vi "Get Database Items.vi"(6 "bookable":bool, 7 "search string":string, 8 "error in (no error)":errorcluster, 9 "offset (0)":u32, 10 "limit (15)":u32=15, 11 "eLab in":refnum<class "PL eLabFTW Client.lvclass">) -> (0 "error out":errorcluster, 2 "database items":T1(array[cluster]) {"last comment"."datetime" format="%<%X\n%x>T"; "last change"."datetime" format="%<%X\n%x>T"; "start datetime" format="%<%X\n%x>T"}, 3 "eLab out":refnum<class "PL eLabFTW Client.lvclass">)   [LabVIEW 2015, in "PL eLabFTW Client.lvclass"]
doc: "Gets database items. Limit, offset and search string can be used to narrow down the output."
uses:
  PL eLabFTW Client.lvclass
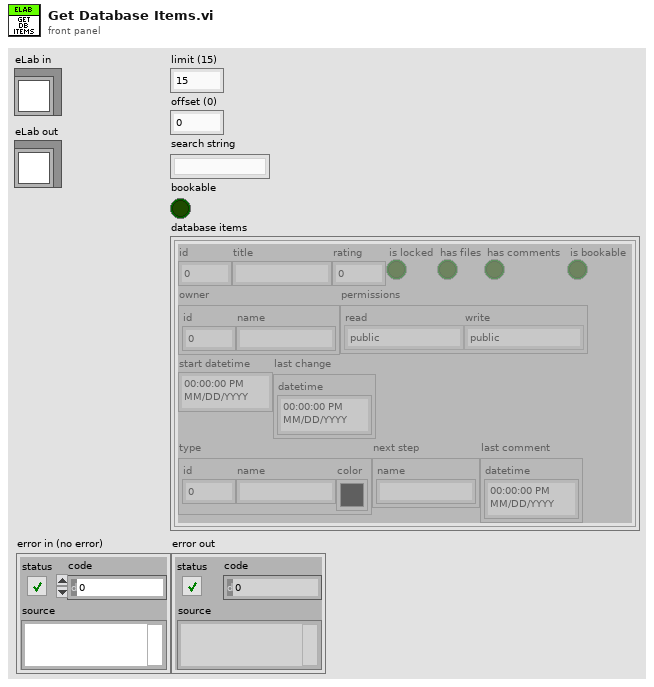
[diagram p1: front panel]
types:
  T1 = cluster{"id":u32, "title":string, "rating":u32, "is locked":bool, "has files":bool, "has comments":bool, "is bookable":bool, "owner":cluster{"id":u32, "name":string}, "permissions":cluster{"read":enum16{"public", "organization", "team", "owner and admins", "owner"}, "write":enum16{"public", "organization", "team", "owner and admins", "owner"}}, "start datetime":timestamp, "last change":cluster{"datetime":timestamp}, "type":cluster{"id":u32, "name":string, "color":u32}, "next step":cluster{"name":string}, "last comment":cluster{"datetime":timestamp}}[]
  T2 = cluster{"id":string, "title":string, "date":string, "category":string, "rating":string, "userid":string, "locked":string, "canread":string, "canwrite":string, "lastchange":string, "up_item_id":string, "has_attachment":string, "next_step":string, "category_id":string, "color":string, "fullname":string, "recent_comment":string, "has_comment":string, "bookable":string}[]
  T3 = cluster{"id":u32, "title":string, "rating":u32, "is locked":bool, "has files":bool, "has comments":bool, "is bookable":bool, "owner":cluster{"id":u32, "name":string}, "permissions":cluster{"read":enum16{"public", "organization", "team", "owner and admins", "owner"}, "write":enum16{"public", "organization", "team", "owner and admins", "owner"}}, "start datetime":timestamp, "last change":cluster{"datetime":timestamp}, "type":cluster{"id":u32, "name":string, "color":u32}, "next step":cluster{"name":string}, "last comment":cluster{"datetime":timestamp}}
  T4 = enum16{"public", "organization", "team", "owner and admins", "owner"}
  T5 = cluster{"id":i32, "title":i32, "date":i32, "category":i32, "rating":i32, "userid":i32, "locked":i32, "canread":i32, "canwrite":i32, "lastchange":i32, "up_item_id":i32, "has_attachment":i32, "next_step":i32, "category_id":i32, "color":i32, "fullname":i32, "recent_comment":i32, "has_comment":i32, "bookable":i32}
  T6 = cluster{"id":bool, "title":bool, "date":bool, "category":bool, "rating":bool, "userid":bool, "locked":bool, "canread":bool, "canwrite":bool, "lastchange":bool, "up_item_id":bool, "has_attachment":bool, "next_step":bool, "category_id":bool, "color":bool, "fullname":bool, "recent_comment":bool, "has_comment":bool, "bookable":bool}
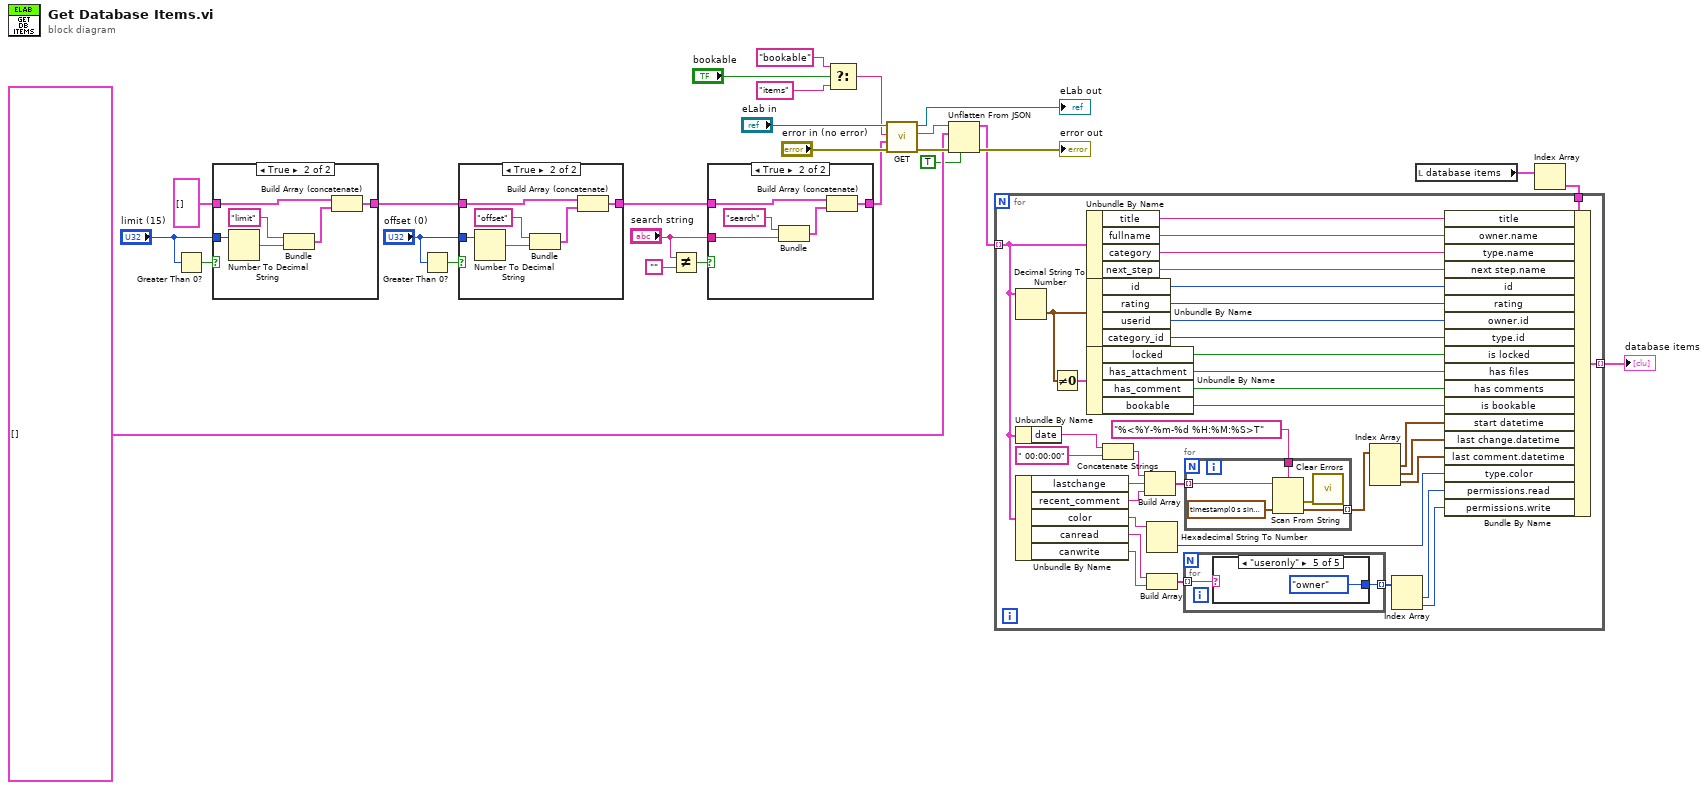
[diagram p0: block diagram]
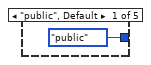
[diagram p2: hidden frame]
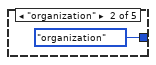
[diagram p3: hidden frame]
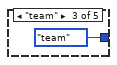
[diagram p4: hidden frame]
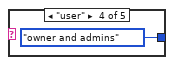
[diagram p5: hidden frame]
diagram:
  n1 = Greater Than 0?(x="limit (15)") -> (x > 0?=w21:bool)
  n2 = case shown="True" w21 {
    tunnel: "limit (15)" -> [_ w34]
    tunnel: [w28 w30] -> w16
    tunnel: cluster{string, string}[] [] -> [w28 w29]
    frame False {
    }
    frame True {
      n3 = Number To Decimal String(number=w34) -> (decimal integer string=w33:string)  [unwired: 1 in]
      n4 = Bundle("limit", w33) -> (w31:cluster{string, string})  [unwired: 1 in]
      n5 = Build Array (concatenate)(w29, w31) -> (w30:cluster{string, string}[])
    }
  }
  n6 = Greater Than 0?(x="offset (0)") -> (x > 0?=w18:bool)
  n7 = case shown="True" w18 {
    tunnel: "offset (0)" -> [_ w41]
    tunnel: [w35 w37] -> w14
    tunnel: w16 -> [w35 w36]
    frame False {
    }
    frame True {
      n8 = Number To Decimal String(number=w41) -> (decimal integer string=w40:string)  [unwired: 1 in]
      n9 = Bundle("offset", w40) -> (w38:cluster{string, string})  [unwired: 1 in]
      n10 = Build Array (concatenate)(w36, w38) -> (w37:cluster{string, string}[])
    }
  }
  n11 = Not Equal?(x="search string", y="") -> (x != y?=w15:bool)
  n12 = case shown="True" w15 {
    tunnel: "search string" -> [_ w43]
    tunnel: [w42 w45] -> w10
    tunnel: w14 -> [w42 w44]
    frame False {
    }
    frame True {
      n13 = Bundle("search", "search string"=w43) -> (w46:cluster{string, "search string":string})  [unwired: 1 in]
      n14 = Build Array (concatenate)(w44, w46) -> (w45:cluster{string, "search string":string}[])
    }
  }
  n15 = Select(t="bookable" ("relative URL"), s="bookable", f="items" ("relative URL")) -> (s? t:f=w1:string)
  n16 = call "GET.vi"("error in (no error)"="error in (no error)", "parameters"=w10, "relative URL"=w1, "eLab in"="eLab in") -> ("error out"=w24:errorcluster, "response body"=w7:string, "eLab out"=→"eLab out":refnum<class "PL eLabFTW Client.lvclass">)  [unwired: 5 in]
  n17 = Unflatten From JSON(JSON string=w7, type and defaults=T2 [], default null elements? (F)=TRUE, error in (no error)=w24) -> (value=w22:T2, error out=→"error out":errorcluster)  [unwired: 3 in]
  n18 = local read "database items"() -> (w9:T1)
  n19 = Index Array(array=w9) -> (element=w8:T3)  [unwired: 1 in]
  n20 = for {
    tunnel: w22 -> [w54] mode=indexing
    tunnel: w8 -> [w49]
    tunnel: [w70] -> w5 mode=indexing
    n21 = Decimal String To Number(string=w54) -> (number=w75:T5)  [unwired: 2 in, 1 out]
    n22 = Unbundle By Name(w54) -> ("date"=w52:string)
    n23 = Unbundle By Name(w54) -> ("lastchange"=w68:string, "recent_comment"=w69:string, "color"=w63:string, "canread"=w61:string, "canwrite"=w60:string)
    n24 = Not Equal To 0?(x=w75) -> (x != 0?=w74:T6)
    n25 = Unbundle By Name(w54) -> ("title"=w83:string, "fullname"=w82:string, "category"=w81:string, "next_step"=w80:string)
    n26 = Unbundle By Name(w75) -> ("id"=w79:i32, "rating"=w78:i32, "userid"=w77:i32, "category_id"=w76:i32)
    n27 = Unbundle By Name(w74) -> ("locked"=w73:bool, "has_attachment"=w72:bool, "has_comment"=w71:bool, "bookable"=w48:bool)
    n28 = Concatenate Strings(w52, " 00:00:00" ("string")) -> (w51:string)
    n29 = Build Array(w51, w68, w69) -> (w67:string[])
    n30 = Hexadecimal String To Number(string=w63) -> (number=w62:u32)  [unwired: 2 in, 1 out]
    n31 = Build Array(w61, w60) -> (w59:string[])
    n32 = for {
      tunnel: w59 -> [w85] mode=indexing
      tunnel: [w84] -> w58 mode=indexing
      n33 = case shown="\"useronly\"" w85 {
        tunnel: [T4."public" ("permissions.read") T4."organization" ("permissions.read") T4."team" ("permissions.read") T4."owner and admins" ("permissions.read") T4."owner" ("permissions.read")] -> w84
        frame "public", Default {
        }
        frame "organization" {
        }
        frame "team" {
        }
        frame "user" {
        }
        frame "useronly" {
        }
      }
    }
    n34 = for {
      tunnel: w67 -> [w93] mode=indexing
      tunnel: [w92] -> w66 mode=indexing
      tunnel: "%<%Y-%m-%d %H:%M:%S>T" ("format string") -> [w91]
      n35 = Scan From String(format string=w91, input string=w93, default 1=timestamp(0 s since 1904-01-01) ("from")) -> (error out=w95:errorcluster, output 1=w92:timestamp)  [unwired: 2 in, 2 out]
      n36 = call <vilib>:"Clear Errors.vi"("error in (no error)"=w95) -> ()  [unwired: 5 in, 2 out]
    }
    n37 = Index Array(array=w66) -> (element #1=w53:timestamp, element #2=w65:timestamp, element #3=w64:timestamp)  [unwired: 3 in]
    n38 = Index Array(array=w58) -> (element #1=w57:T4, element #2=w56:T4)  [unwired: 2 in]
    n39 = Bundle By Name(cluster=w49, "title"=w83, "owner.name"=w82, "type.name"=w81, "next step.name"=w80, "id"=w79, "rating"=w78, "owner.id"=w77, "type.id"=w76, "is locked"=w73, "has files"=w72, "has comments"=w71, "is bookable"=w48, "start datetime"=w53, "last change.datetime"=w65, "last comment.datetime"=w64, "type.color"=w62, "permissions.read"=w57, "permissions.write"=w56) -> (w70:T3)
  }
  "database items" <- w5
